vi "Target Initialize Variables.vi"() -> (0 "Error Out":errorcluster)   [LabVIEW 2018]
uses:
  COBRA-Libraries/Data Logging/File Headers Array.ctl
  COBRA-Libraries/Data Logging/Target Metadata Headers Array.ctl
  COBRA-Libraries/Data Logging/COBRA Logging and Loop Timing Library.lvlib
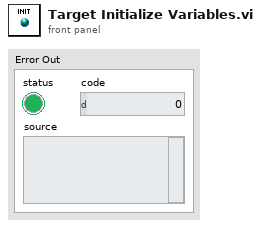
[diagram p1: front panel]
types:
  T1 = typedef "COBRA Logging and Loop Timing Library.lvlib/Target Metadata Headers Array.ctl" = string[]
  T2 = typedef "COBRA Logging and Loop Timing Library.lvlib/File Headers Array.ctl" = string[]
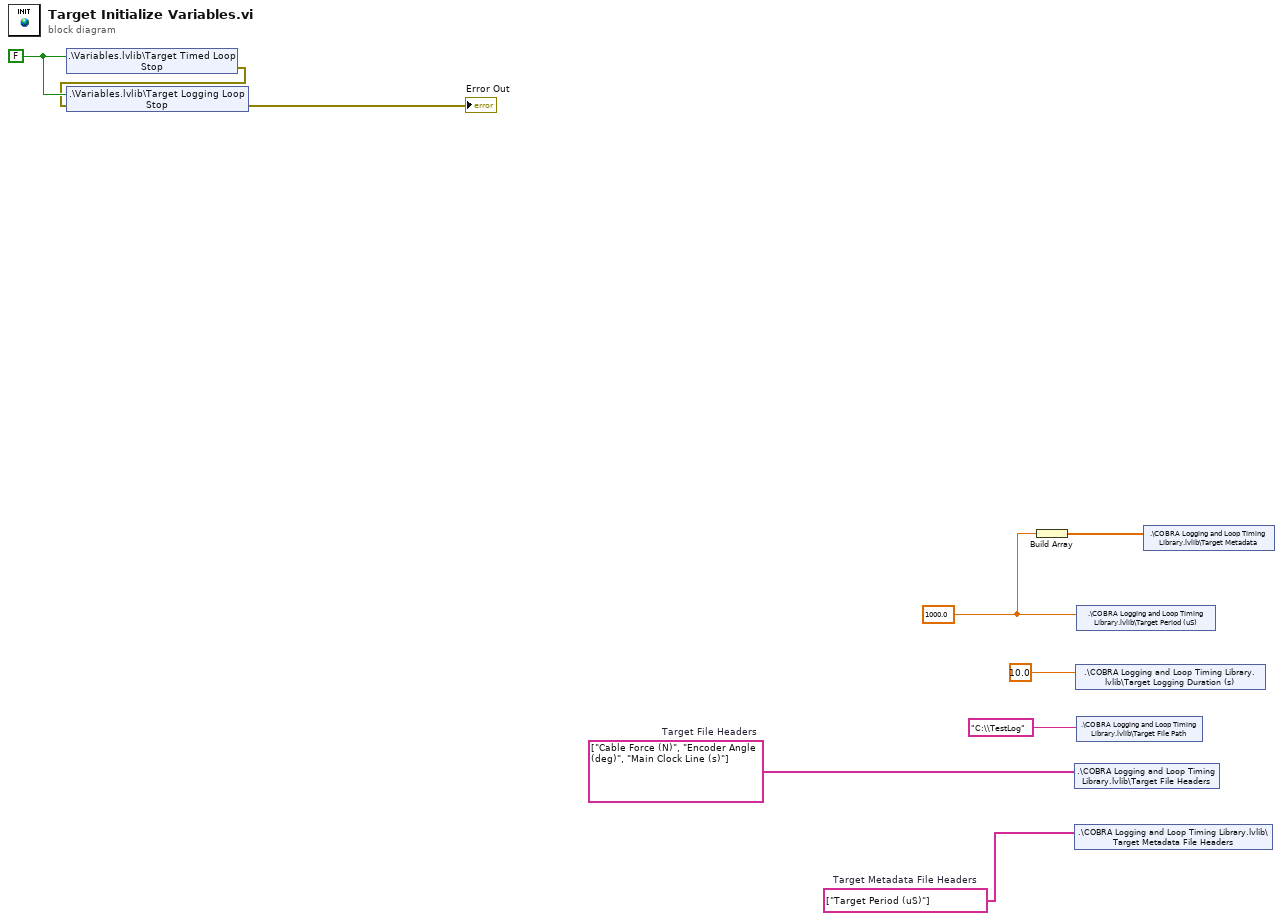
[diagram p0: block diagram]
diagram:
  w2 = T1 ["Target Period (uS)"]  # Target Metadata File Headers
  w1 = T2 ["Cable Force (N)", "Encoder Angle (deg)", "Main Clock Line (s)"]  # Target File Headers
  w5 = 1000.0 ("Target Period (uS)")
  w9 = FALSE ("PXI Timed Loop Stop")
  n1 = shared-variable ".\\Variables.lvlib\\Target Timed Loop Stop"(w9) -> (error out=w8:errorcluster)  [unwired: 1 in]
  n2 = shared-variable ".\\Variables.lvlib\\Target Logging Loop Stop"(w9, error in=w8) -> (error out=→"Error Out":errorcluster)
  n3 = Build Array(w5) -> (w6:dbl[])
  n4 = shared-variable ".\\COBRA Logging and Loop Timing Library.lvlib\\Target File Headers"(w1) -> ()  [unwired: 1 in, 1 out]
  n5 = shared-variable ".\\COBRA Logging and Loop Timing Library.lvlib\\Target Metadata File Headers"(w2) -> ()  [unwired: 1 in, 1 out]
  n6 = shared-variable ".\\COBRA Logging and Loop Timing Library.lvlib\\Target Logging Duration (s)"(10.0 ("Target Logging Duration (s)")) -> ()  [unwired: 1 in, 1 out]
  n7 = shared-variable ".\\COBRA Logging and Loop Timing Library.lvlib\\Target Period (uS)"(w5) -> ()  [unwired: 1 in, 1 out]
  n8 = shared-variable ".\\COBRA Logging and Loop Timing Library.lvlib\\Target File Path"("C:\\TestLog" ("Target File Path")) -> ()  [unwired: 1 in, 1 out]
  n9 = shared-variable ".\\COBRA Logging and Loop Timing Library.lvlib\\Target Metadata"(w6) -> ()  [unwired: 1 in, 1 out]
